vi "fxpInit.vi"(3 "Container State":T8, 4 "Previous State":variant, 5 "Previous Version":T7) -> (2 "Current State":T1)   [LabVIEW 2020, in "FXP.xctl"]
uses:
  <vilib>/fxp/FXPxcontrol/FXP.xctl
  <vilib>/fxp/FXPxcontrol/fxpState.ctl
  <vilib>/fxp/LVFixedPointQuantizationPolicyTypeDef.ctl
  <vilib>/fxp/LVFixedPointOverflowPolicyTypeDef.ctl
  <vilib>/fxp/FXPxcontrol/fxpChangeEvent.ctl
  <vilib>/fxp/FXPxcontrol/fxpValueChangeControl.ctl
  <vilib>/fxp/FXPxcontrol/fxpMixedStateStatus.ctl
  <vilib>/_xctls/Container State.ctl
  <vilib>/_xctls/Version.ctl
  <vilib>/_xctls/XControlSupport.lvlib
panel:
  in  "Default Indicator State":T1
  in  "Default Control State":T1
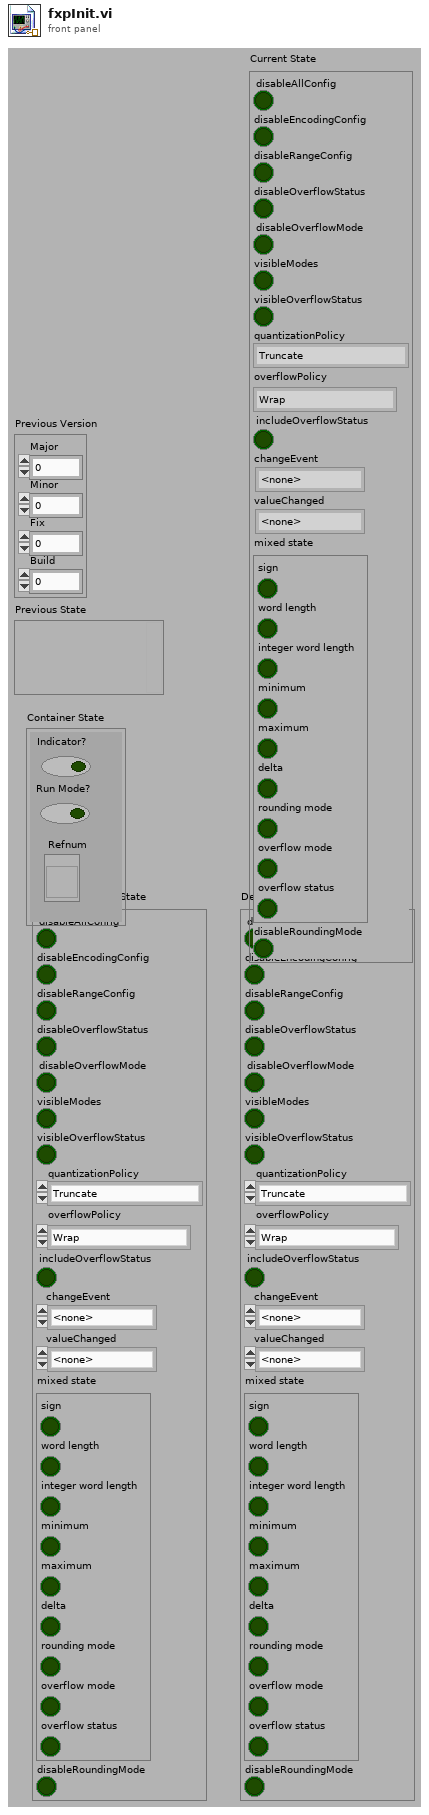
[diagram p1: front panel]
types:
  T1 = typedef "FXP.xctl/fxpState.ctl" = cluster{"disableAllConfig":bool, "disableEncodingConfig":bool, "disableRangeConfig":bool, "disableOverflowStatus":bool, "disableOverflowMode":bool, "visibleModes":bool, "visibleOverflowStatus":bool, "quantizationPolicy":T2, "overflowPolicy":T3, "includeOverflowStatus":bool, "changeEvent":T4, "valueChanged":T5, "mixed state":T6, "disableRoundingMode":bool}
  T2 = typedef "LVFixedPointQuantizationPolicyTypeDef.ctl" = enum32{"Truncate", "Round-Half-Up (Asymmetric)", "Round-Half-Even"}
  T3 = typedef "LVFixedPointOverflowPolicyTypeDef.ctl" = enum32{"Wrap", "Saturate"}
  T4 = typedef "FXP.xctl/fxpChangeEvent.ctl" = enum16{"<none>", "initialize", "modesVisible", "overflowModeEnabled", "overflowStatusVisible", "configEnabled", "modeRounding", "modeOverflow", "statusOverflow", "mixedState", "roundingModeEnabled"}
  T5 = typedef "FXP.xctl/fxpValueChangeControl.ctl" = enum16{"<none>", "sign", "word length", "integer word length", "minimum", "maximum", "delta", "rounding mode", "overflow mode", "overflow status"}
  T6 = typedef "FXP.xctl/fxpMixedStateStatus.ctl" = cluster{"sign":bool, "word length":bool, "integer word length":bool, "minimum":bool, "maximum":bool, "delta":bool, "rounding mode":bool, "overflow mode":bool, "overflow status":bool}
  T7 = typedef "XControlSupport.lvlib/Version.ctl" = cluster{"Major":u16, "Minor":u16, "Fix":u16, "Build":u16}
  T8 = typedef "XControlSupport.lvlib/Container State.ctl" = cluster{"Indicator?":bool, "Run Mode?":bool, " Refnum":refnum<vi>}
  T9 = cluster{"enableTypeConfig":bool, "visibleModes":bool, "quantizationPolicy":u32, "overflowPolicy":u32, "changeEvent":u16, "rangeChanged":bool}
  T10 = cluster{"enableTypeConfig":bool, "visibleModes":bool, "visibleOverflowStatus":bool, "quantizationPolicy":u32, "overflowPolicy":u32, "includeOverflowStatus":bool, "changeEvent":u16, "valueChanged":u16, "mixed state":cluster{"sign":bool, "word length":bool, "integer word length":bool, "minimum":bool, "maximum":bool, "delta":bool, "rounding mode":bool, "overflow mode":bool, "overflow status":bool}}
  T11 = cluster{"sign":bool, "word length":bool, "integer word length":bool, "minimum":bool, "maximum":bool, "delta":bool, "rounding mode":bool, "overflow mode":bool, "overflow status":bool}
  T12 = cluster{"enableTypeConfig":bool, "visibleModes":bool, "visibleOverflowStatus":bool, "quantizationPolicy":u32, "overflowPolicy":u32, "includeOverflowStatus":bool, u16, u16, "mixed state":cluster{"sign":bool, "word length":bool, "integer word length":bool, "minimum":bool, "maximum":bool, "delta":bool, "rounding mode":bool, "overflow mode":bool, "overflow status":bool}}
  T13 = cluster{"enableTypeConfig":bool, "visibleModes":bool, "enableOverflowMode":bool, "visibleOverflowStatus":bool, "quantizationPolicy":u32, "overflowPolicy":u32, "includeOverflowStatus":bool, u16, u16, "mixed state":cluster{"sign":bool, "word length":bool, "integer word length":bool, "minimum":bool, "maximum":bool, "delta":bool, "rounding mode":bool, "overflow mode":bool, "overflow status":bool}}
  T14 = cluster{"disableEncodingConfig":bool, "disableRangeConfig":bool, "disableOverflowStatus":bool, "disableOverflowMode":bool, "visibleModes":bool, "visibleOverflowStatus":bool, "quantizationPolicy":u32, "overflowPolicy":u32, "includeOverflowStatus":bool, u16, u16, "mixed state":cluster{"sign":bool, "word length":bool, "integer word length":bool, "minimum":bool, "maximum":bool, "delta":bool, "rounding mode":bool, "overflow mode":bool, "overflow status":bool}}
  T15 = cluster{"disableAllConfig":bool, "disableEncodingConfig":bool, "disableRangeConfig":bool, "disableOverflowStatus":bool, "disableOverflowMode":bool, "visibleModes":bool, "visibleOverflowStatus":bool, "quantizationPolicy":enum32{"Truncate", "Round-Half-Up (Asymmetric)", "Round-Half-Even"}, "overflowPolicy":enum32{"Wrap", "Saturate"}, "includeOverflowStatus":bool, "changeEvent":enum16{"<none>", "initialize", "modesVisible", "overflowModeEnabled", "overflowStatusVisible", "configEnabled", "modeRounding", "modeOverflow", "statusOverflow", "mixedState"}, "valueChanged":enum16{"<none>", "sign", "word length", "integer word length", "minimum", "maximum", "delta", "rounding mode", "overflow mode", "overflow status"}, "mixed state":cluster{"sign":bool, "word length":bool, "integer word length":bool, "minimum":bool, "maximum":bool, "delta":bool, "rounding mode":bool, "overflow mode":bool, "overflow status":bool}}
  T16 = enum32{"Truncate", "Round-Half-Up (Asymmetric)", "Round-Half-Even"}
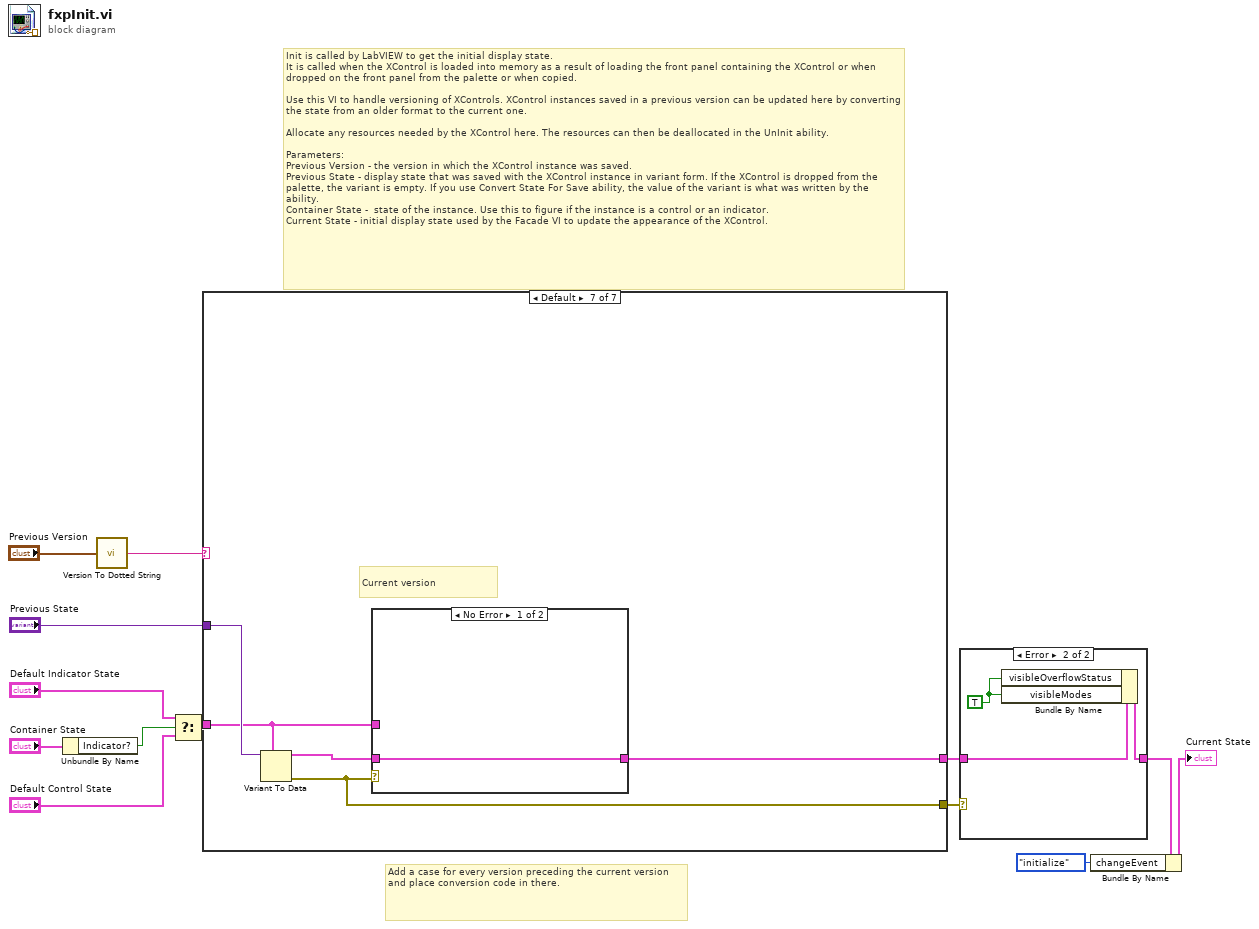
[diagram p0: block diagram]
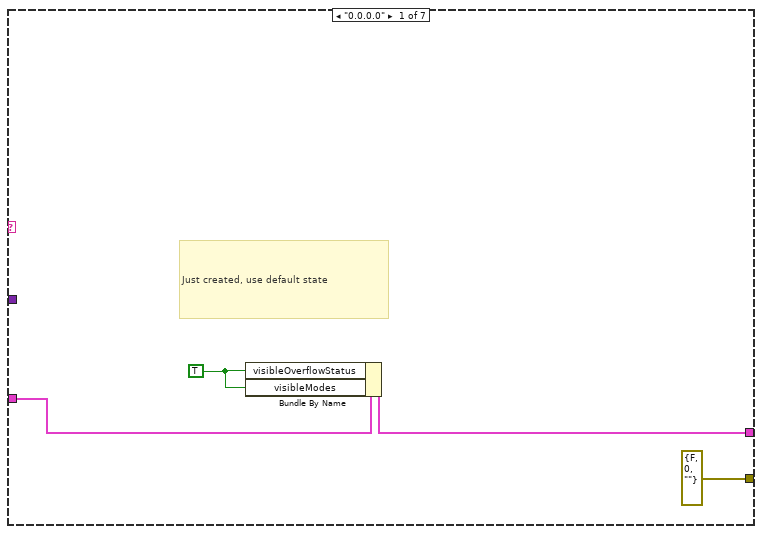
[diagram p3: hidden frame]
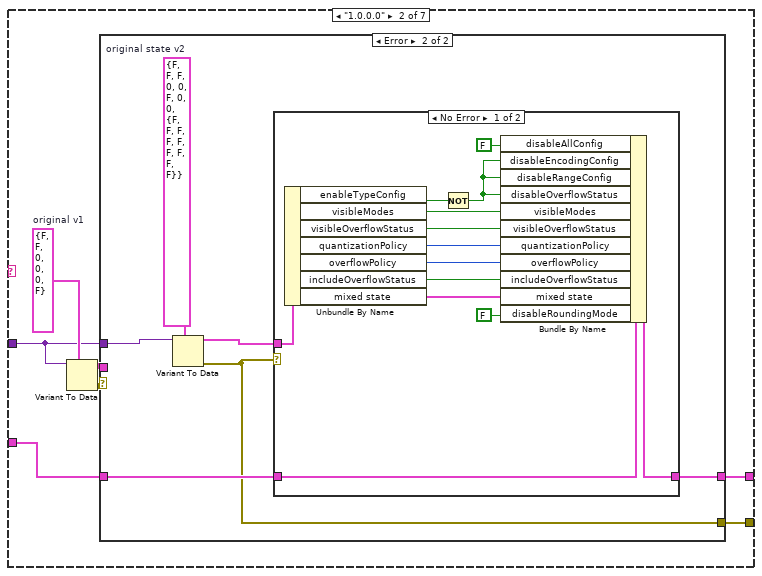
[diagram p4: hidden frame]
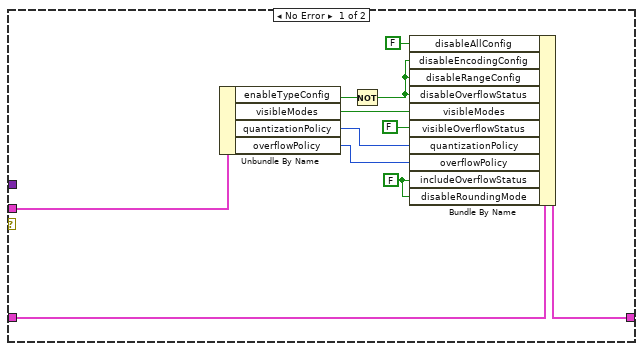
[diagram p5: hidden frame]
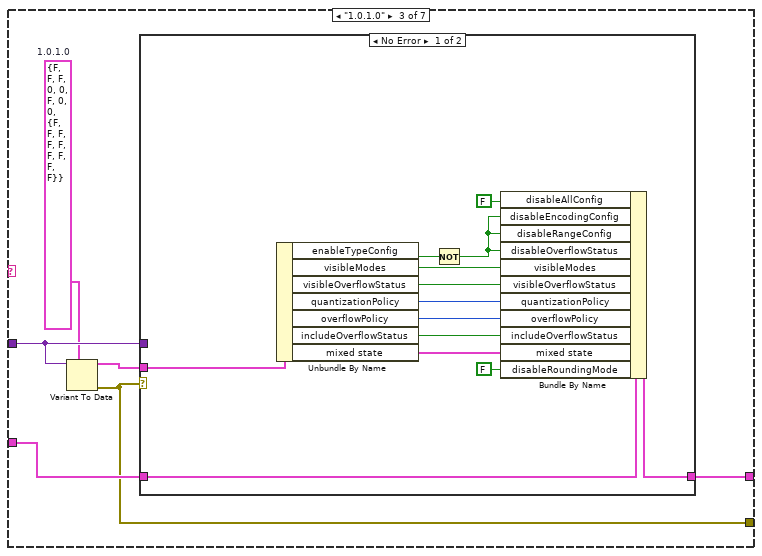
[diagram p7: hidden frame]
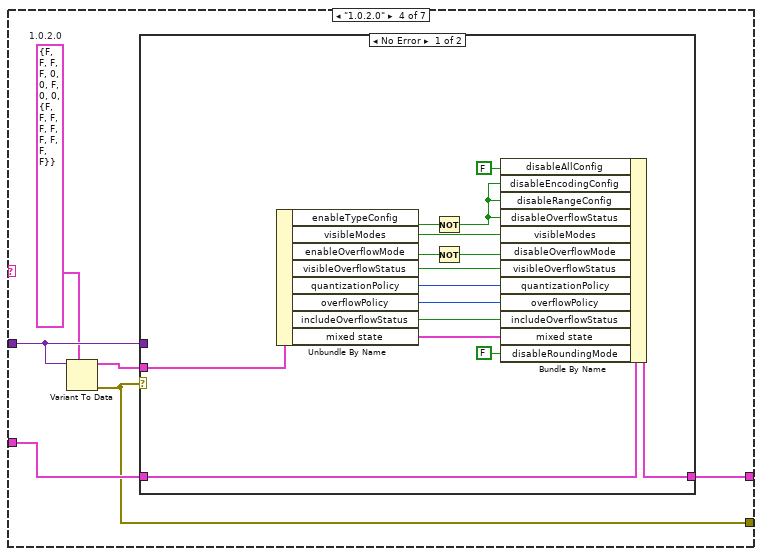
[diagram p9: hidden frame]
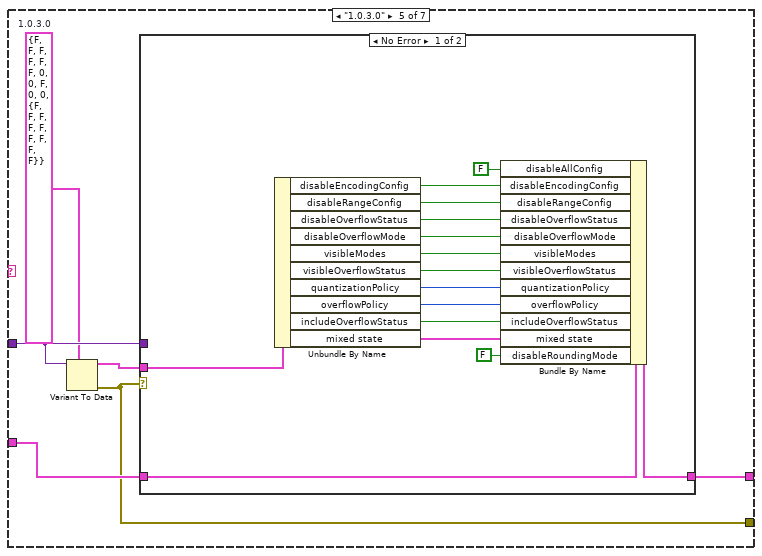
[diagram p11: hidden frame]
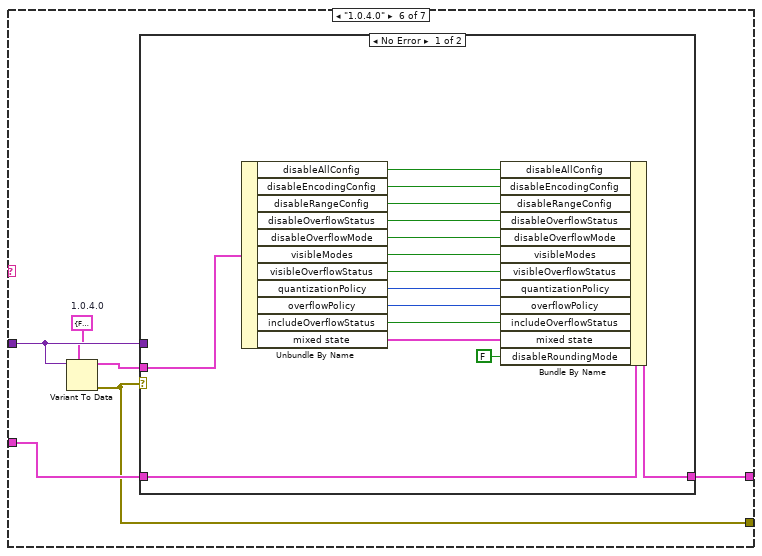
[diagram p13: hidden frame]
diagram:
  # "Add a case for every version preceding the current version and place conversion code in there."
  # "Init is called by LabVIEW to get the initial display state.\nIt is called when the XControl is loaded into memory as a result of loading the front panel containing the XControl or when dropped on the front panel from the palette or when copied.\n\nUse this VI to handle versioning of XControls. XControl instances saved in a previous version can be updated here by converting the state from an older format to the current one.\n\nAllocate any resources needed by the XControl here. The resources can then be deallocated in the UnInit ability.\n\nParameters:\nPrevious Version - the version in which the XControl instance was saved.\nPrevious State - display state that was saved with the XControl instance in variant form. If the XControl is dropped from the palette, the variant is empty. If you use Convert State For Save ability, the value of the variant is what was written by the ability. \nContainer State -  state of the instance. Use this to figure if the instance is a control or an indicator.\nCurrent State - initial display state used by the Facade VI to update the appearance of the XControl."
  n1 = Unbundle By Name("Container State") -> ("Indicator?"=w9:bool)
  n2 = call <vilib>:"Version To Dotted String.vi"("Version"="Previous Version") -> ("String Version"=w6:string)
  n3 = Select(t="Default Indicator State", s=w9, f="Default Control State") -> (s? t:f=w8:T1)
  n4 = case shown="Default" w6 {
    tunnel: "Previous State" -> [_ w19 w58 w78 w100 w122 w146]
    tunnel: [w16 w23 w60 w80 w102 w124 w143] -> w4
    tunnel: w8 -> [w17 w24 w61 w81 w103 w125 w144]
    tunnel: [errorcluster {"status"=FALSE, "code"=0, "source"=""} ("error out") w18 w56 w76 w99 w121 w142] -> w5
    frame "0.0.0.0" {
      w14 = TRUE ("enableTypeConfig")
      # "Just created, use default state"
      n5 = Bundle By Name(cluster=w17, "visibleOverflowStatus"=w14, "visibleModes"=w14) -> (w16:T1)
    }
    frame "1.0.0.0" {
      w22 = T9 {"enableTypeConfig"=FALSE, "visibleModes"=FALSE, "quantizationPolicy"=0, "overflowPolicy"=0, "changeEvent"=0, "rangeChanged"=FALSE}  # original v1
      n6 = Variant To Data(type=w22, Variant=w19) -> (data=w20:T9, error out=w21:errorcluster)  [unwired: 1 in]
      n7 = case shown="Error" w21 {
        tunnel: w24 -> [w35 w41]
        tunnel: [w34 w40] -> w23
        tunnel: w20 -> [w33 _]
        tunnel: w19 -> [_ w39]
        tunnel: [_ w36] -> w18
        frame No Error {
          w26 = FALSE ("enableOverflowMode")
          n8 = Unbundle By Name(w33) -> ("enableTypeConfig"=w32:bool, "visibleModes"=w25:bool, "quantizationPolicy"=w30:u32, "overflowPolicy"=w29:u32)
          n9 = Not(x=w32) -> (.not. x?=w28:bool)
          n10 = Bundle By Name(cluster=w35, "disableAllConfig"=FALSE, "disableEncodingConfig"=w28, "disableRangeConfig"=w28, "disableOverflowStatus"=w28, "visibleModes"=w25, "visibleOverflowStatus"=FALSE, "quantizationPolicy"=w30, "overflowPolicy"=w29, "includeOverflowStatus"=w26, "disableRoundingMode"=w26) -> (w34:T1)
        }
        frame Error {
          w38 = T10 {"enableTypeConfig"=FALSE, "visibleModes"=FALSE, "visibleOverflowStatus"=FALSE, "quantizationPolicy"=0, "overflowPolicy"=0, "includeOverflowStatus"=FALSE, "changeEvent"=0, "valueChanged"=0, "mixed state"={"sign"=FALSE, "word length"=FALSE, "integer word length"=FALSE, "minimum"=FALSE, "maximum"=FALSE, "delta"=FALSE, "rounding mode"=FALSE, "overflow mode"=FALSE, "overflow status"=FALSE}}  # original state v2
          n11 = Variant To Data(type=w38, Variant=w39) -> (data=w37:T10, error out=w36:errorcluster)  [unwired: 1 in]
          n12 = case shown="No Error" w36 {
            tunnel: w41 -> [w54 w55]
            tunnel: [w53 w55] -> w40
            tunnel: w37 -> [w52 _]
            frame No Error {
              n13 = Unbundle By Name(w52) -> ("enableTypeConfig"=w51:bool, "visibleModes"=w43:bool, "visibleOverflowStatus"=w50:bool, "quantizationPolicy"=w49:u32, "overflowPolicy"=w48:u32, "includeOverflowStatus"=w47:bool, "mixed state"=w46:T11)
              n14 = Not(x=w51) -> (.not. x?=w45:bool)
              n15 = Bundle By Name(cluster=w54, "disableAllConfig"=FALSE, "disableEncodingConfig"=w45, "disableRangeConfig"=w45, "disableOverflowStatus"=w45, "visibleModes"=w43, "visibleOverflowStatus"=w50, "quantizationPolicy"=w49, "overflowPolicy"=w48, "includeOverflowStatus"=w47, "mixed state"=w46, "disableRoundingMode"=FALSE) -> (w53:T1)
            }
            frame Error {
            }
          }
        }
      }
    }
    frame "1.0.1.0" {
      w57 = T12 {"enableTypeConfig"=FALSE, "visibleModes"=FALSE, "visibleOverflowStatus"=FALSE, "quantizationPolicy"=0, "overflowPolicy"=0, "includeOverflowStatus"=FALSE, 0, 0, "mixed state"={"sign"=FALSE, "word length"=FALSE, "integer word length"=FALSE, "minimum"=FALSE, "maximum"=FALSE, "delta"=FALSE, "rounding mode"=FALSE, "overflow mode"=FALSE, "overflow status"=FALSE}}  # 1.0.1.0
      n16 = Variant To Data(type=w57, Variant=w58) -> (data=w59:T12, error out=w56:errorcluster)  [unwired: 1 in]
      n17 = case shown="No Error" w56 {
        tunnel: w61 -> [w74 w75]
        tunnel: [w73 w75] -> w60
        tunnel: w59 -> [w72 _]
        tunnel: w58 -> [_ _]
        frame No Error {
          n18 = Unbundle By Name(w72) -> ("enableTypeConfig"=w71:bool, "visibleModes"=w62:bool, "visibleOverflowStatus"=w67:bool, "quantizationPolicy"=w70:u32, "overflowPolicy"=w69:u32, "includeOverflowStatus"=w68:bool, "mixed state"=w66:T11)
          n19 = Not(x=w71) -> (.not. x?=w65:bool)
          n20 = Bundle By Name(cluster=w74, "disableAllConfig"=FALSE, "disableEncodingConfig"=w65, "disableRangeConfig"=w65, "disableOverflowStatus"=w65, "visibleModes"=w62, "visibleOverflowStatus"=w67, "quantizationPolicy"=w70, "overflowPolicy"=w69, "includeOverflowStatus"=w68, "mixed state"=w66, "disableRoundingMode"=FALSE) -> (w73:T1)
        }
        frame Error {
        }
      }
    }
    frame "1.0.2.0" {
      w77 = T13 {"enableTypeConfig"=FALSE, "visibleModes"=FALSE, "enableOverflowMode"=FALSE, "visibleOverflowStatus"=FALSE, "quantizationPolicy"=0, "overflowPolicy"=0, "includeOverflowStatus"=FALSE, 0, 0, "mixed state"={"sign"=FALSE, "word length"=FALSE, "integer word length"=FALSE, "minimum"=FALSE, "maximum"=FALSE, "delta"=FALSE, "rounding mode"=FALSE, "overflow mode"=FALSE, "overflow status"=FALSE}}  # 1.0.2.0
      n21 = Variant To Data(type=w77, Variant=w78) -> (data=w79:T13, error out=w76:errorcluster)  [unwired: 1 in]
      n22 = case shown="No Error" w76 {
        tunnel: w81 -> [w96 w97]
        tunnel: [w95 w97] -> w80
        tunnel: w79 -> [w94 _]
        tunnel: w78 -> [_ _]
        frame No Error {
          n23 = Unbundle By Name(w94) -> ("enableTypeConfig"=w93:bool, "visibleModes"=w83:bool, "enableOverflowMode"=w88:bool, "visibleOverflowStatus"=w89:bool, "quantizationPolicy"=w92:u32, "overflowPolicy"=w91:u32, "includeOverflowStatus"=w90:bool, "mixed state"=w86:T11)
          n24 = Not(x=w93) -> (.not. x?=w85:bool)
          n25 = Not(x=w88) -> (.not. x?=w87:bool)
          n26 = Bundle By Name(cluster=w96, "disableAllConfig"=FALSE, "disableEncodingConfig"=w85, "disableRangeConfig"=w85, "disableOverflowStatus"=w85, "visibleModes"=w83, "disableOverflowMode"=w87, "visibleOverflowStatus"=w89, "quantizationPolicy"=w92, "overflowPolicy"=w91, "includeOverflowStatus"=w90, "mixed state"=w86, "disableRoundingMode"=FALSE) -> (w95:T1)
        }
        frame Error {
        }
      }
    }
    frame "1.0.3.0" {
      w98 = T14 {"disableEncodingConfig"=FALSE, "disableRangeConfig"=FALSE, "disableOverflowStatus"=FALSE, "disableOverflowMode"=FALSE, "visibleModes"=FALSE, "visibleOverflowStatus"=FALSE, "quantizationPolicy"=0, "overflowPolicy"=0, "includeOverflowStatus"=FALSE, 0, 0, "mixed state"={"sign"=FALSE, "word length"=FALSE, "integer word length"=FALSE, "minimum"=FALSE, "maximum"=FALSE, "delta"=FALSE, "rounding mode"=FALSE, "overflow mode"=FALSE, "overflow status"=FALSE}}  # 1.0.3.0
      n27 = Variant To Data(type=w98, Variant=w100) -> (data=w101:T14, error out=w99:errorcluster)  [unwired: 1 in]
      n28 = case shown="No Error" w99 {
        tunnel: w103 -> [w118 w119]
        tunnel: [w117 w119] -> w102
        tunnel: w101 -> [w116 _]
        tunnel: w100 -> [_ _]
        frame No Error {
          n29 = Unbundle By Name(w116) -> ("disableEncodingConfig"=w110:bool, "disableRangeConfig"=w109:bool, "disableOverflowStatus"=w108:bool, "disableOverflowMode"=w107:bool, "visibleModes"=w104:bool, "visibleOverflowStatus"=w112:bool, "quantizationPolicy"=w115:u32, "overflowPolicy"=w114:u32, "includeOverflowStatus"=w113:bool, "mixed state"=w111:T11)
          n30 = Bundle By Name(cluster=w118, "disableAllConfig"=FALSE, "disableEncodingConfig"=w110, "disableRangeConfig"=w109, "disableOverflowStatus"=w108, "disableOverflowMode"=w107, "visibleModes"=w104, "visibleOverflowStatus"=w112, "quantizationPolicy"=w115, "overflowPolicy"=w114, "includeOverflowStatus"=w113, "mixed state"=w111, "disableRoundingMode"=FALSE) -> (w117:T1)
        }
        frame Error {
        }
      }
    }
    frame "1.0.4.0" {
      w120 = T15 {"disableAllConfig"=FALSE, "disableEncodingConfig"=FALSE, "disableRangeConfig"=FALSE, "disableOverflowStatus"=FALSE, "disableOverflowMode"=FALSE, "visibleModes"=FALSE, "visibleOverflowStatus"=FALSE, "quantizationPolicy"=enum."Truncate", "overflowPolicy"=enum."Wrap", "includeOverflowStatus"=FALSE, "changeEvent"=enum."<none>", "valueChanged"=enum."<none>", "mixed state"={"sign"=FALSE, "word length"=FALSE, "integer word length"=FALSE, "minimum"=FALSE, "maximum"=FALSE, "delta"=FALSE, "rounding mode"=FALSE, "overflow mode"=FALSE, "overflow status"=FALSE}}  # 1.0.4.0
      n31 = Variant To Data(type=w120, Variant=w122) -> (data=w123:T15, error out=w121:errorcluster)  [unwired: 1 in]
      n32 = case shown="No Error" w121 {
        tunnel: w125 -> [w140 w141]
        tunnel: [w139 w141] -> w124
        tunnel: w123 -> [w138 _]
        tunnel: w122 -> [_ _]
        frame No Error {
          n33 = Unbundle By Name(w138) -> ("disableAllConfig"=w128:bool, "disableEncodingConfig"=w132:bool, "disableRangeConfig"=w131:bool, "disableOverflowStatus"=w130:bool, "disableOverflowMode"=w129:bool, "visibleModes"=w126:bool, "visibleOverflowStatus"=w134:bool, "quantizationPolicy"=w137:T16, "overflowPolicy"=w136:enum32{"Wrap", "Saturate"}, "includeOverflowStatus"=w135:bool, "mixed state"=w133:T11)
          n34 = Bundle By Name(cluster=w140, "disableAllConfig"=w128, "disableEncodingConfig"=w132, "disableRangeConfig"=w131, "disableOverflowStatus"=w130, "disableOverflowMode"=w129, "visibleModes"=w126, "visibleOverflowStatus"=w134, "quantizationPolicy"=w137, "overflowPolicy"=w136, "includeOverflowStatus"=w135, "mixed state"=w133, "disableRoundingMode"=FALSE) -> (w139:T1)
        }
        frame Error {
        }
      }
    }
    frame Default {
      # "Current version"
      n35 = Variant To Data(type=w144, Variant=w146) -> (data=w145:T1, error out=w142:errorcluster)  [unwired: 1 in]
      n36 = case shown="No Error" w142 {
        tunnel: w145 -> [w147 _]
        tunnel: [w147 w148] -> w143
        tunnel: w144 -> [_ w148]
        frame No Error {
        }
        frame Error {
        }
      }
    }
  }
  n37 = case shown="Error" w5 {
    tunnel: [w149 w151] -> w2
    tunnel: w4 -> [w149 w152]
    frame No Error {
    }
    frame Error {
      w150 = TRUE ("visibleOverflowStatus")
      n38 = Bundle By Name(cluster=w152, "visibleOverflowStatus"=w150, "visibleModes"=w150) -> (w151:T1)
    }
  }
  n39 = Bundle By Name(cluster=w2, "changeEvent"=fxpChangeEvent."initialize") -> (→"Current State":T1)
